vi "SubVI 1.vi"(1 "Channel":dbl, 2 "VISA resource name":refnum<visa-resource-name>, 8 "error in (no error)":errorcluster) -> (0 "error out":errorcluster, 9 "Task":string, 10 "Read String":string)   [LabVIEW 2018]
doc: "Use this template to build a VI to use as a subVI."
uses:
  <vilib>/Instr/_visa.llb/VISA Configure Serial Port (Instr).vi
panel:
  in  "String":string
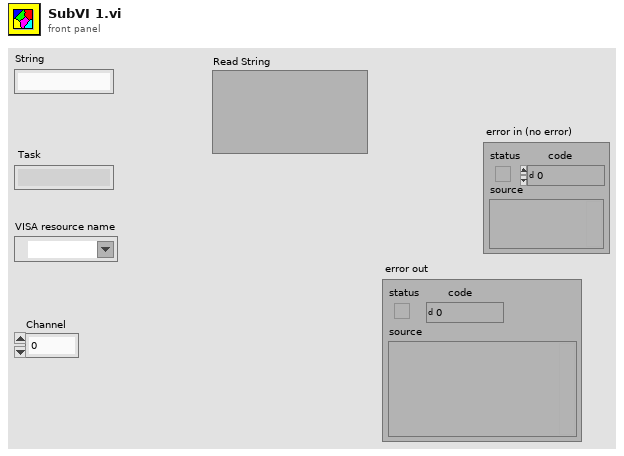
[diagram p1: front panel]
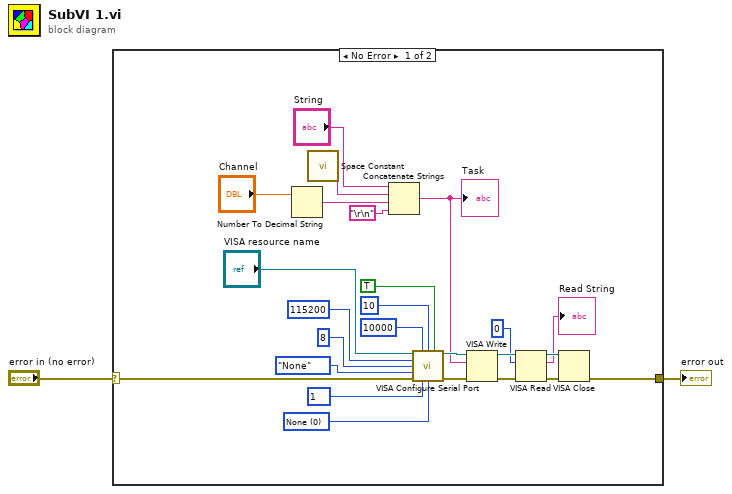
[diagram p0: block diagram]
diagram:
  n1 = case shown="No Error" "error in (no error)" {
    selector: "error in (no error)" -> [w4 w28]
    tunnel: [w3 w28] -> w1
    frame No Error {
      w12 = u16 0 items=["None", "XON/XOFF", "RTS/CTS", "XON/XOFF & RTS/CTS", "DTR/DSR", "XON/XOFF & DTR/DSR"] ("flow control (0:none)")
      w24 = u16 10 items=["1"=10, "1.5"=15, "2.0"=20] ("stop bits (10: 1 bit)")
      n2 = Number To Decimal String(number="Channel") -> (decimal integer string=w5:string)  [unwired: 1 in]
      n3 = call <vilib>:"Space Constant.vi"() -> ("String"=w10:string)
      n4 = Concatenate Strings("String", w10, w5, "\r\n") -> (w7:string)
      "Task" <- w7
      n5 = call-poly "VISA Configure Serial Port"("VISA resource name"="VISA resource name", "timeout (10sec)"=u32 10000, "termination char\n(0xA = '\\n' = LF)"=u8 10 ("termination char\n(0xA = '\\n' = LF)"), "Enable Termination\nChar (T)"=TRUE ("Enable Termination\nChar (T)"), "baud rate (9600)"=115200, "data bits (8)"=8, "parity (0:none)"=enum16{"None", "Odd", "Even", "Mark", "Space"}."None", "error in (no error)"=w4, "stop bits (10: 1 bit)"=w24, "flow control (0:none)"=w12) -> ("VISA resource name out"=w23:refnum<visa-resource-name>, "error out"=w20:errorcluster)  [unwired: 4 in]
      n6 = VISA Write(VISA resource name=w23, write buffer=w7, error in (no error)=w20) -> (VISA resource name out=w22:refnum<visa-resource-name>, error out=w19:errorcluster)  [unwired: 1 out]
      n7 = VISA Read(VISA resource name=w22, byte count=u32 0, error in (no error)=w19) -> (VISA resource name out=w21:refnum<visa-resource-name>, read buffer=→"Read String":string, error out=w18:errorcluster)  [unwired: 1 out]
      n8 = VISA Close(VISA resource name=w21, error in (no error)=w18) -> (error out=w3:errorcluster)
    }
    frame Error {
    }
  }
  "error out" <- w1
